vi "Set_CtlValue.vi"(8 "error in (no error)":errorcluster, 9 "Value":variant, 10 "Control Label":string, 11 "RefCluster In":T1) -> (0 "error out":errorcluster, 3 "RefCluster Out":T1)   [LabVIEW 2020, in "CtlReferences.lvlib" / "CtlReferences.lvclass"]
doc: "This VI uses the GetControlByReference to Set the Value of the specified control as a variant"
uses:
  CtlReferences.lvclass
  TypeDefs/CtlLookup.ctl
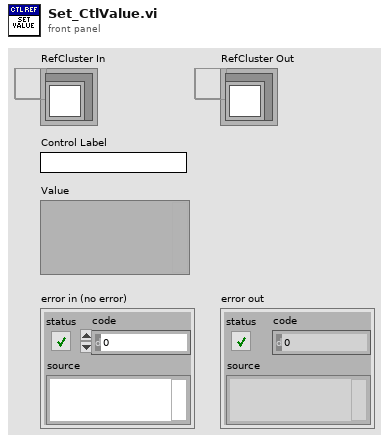
[diagram p1: front panel]
types:
  T1 = typedef "CtlReferences.lvlib/CtlReferences.lvclass/CtlLookup.ctl" = refnum<data-value>
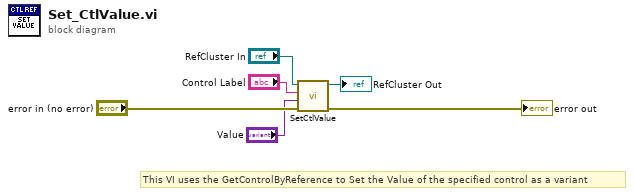
[diagram p0: block diagram]
diagram:
  # "This VI uses the GetControlByReference to Set the Value of the specified control as a variant"
  n1 = call "SetCtlValue.vi"("Error in"="error in (no error)", "Value"="Value", "CtlName In"="Control Label", "CtlLookup In"="RefCluster In") -> ("error out"=→"error out":errorcluster, "CtlLookup Out"=→"RefCluster Out":T1)  [unwired: 6 in]
